vi "Line_Line_Intersection2D_Test_PN.vi"(3 "2D Dir. Vect. of Line 2 (not unit)":dbl[](array[numeric])=[0.0, 0.0], 4 "2D Dir. Vect. of Line 1 (not unit)":dbl[](array[numeric])=[0.0, 0.0], 5 "2D Point on Line 2":dbl[](array[numeric])=[0.0, 0.0], 6 "2D Point on Line 1":dbl[](array[numeric])=[0.0, 0.0]) -> (0 "s2":dbl, 1 "s1":dbl, 2 "Lines Intersect":bool)   [LabVIEW 2011]
panel:
  in  "1+eps":dbl=1.000000000001 format="%#_16f"
  in  "-eps":dbl=-1e-12 format="%#_16f"
  # "The direction vectors must not be unit vectors.\nThe input points must be the tail points of the associated line vectors.\ns1 represents the distance from the start point of line 1 to the intersection point.\ns2 represents the distance from the start point of line 2 to the intersection point."
  # "Paul Nathan 04/03/10"
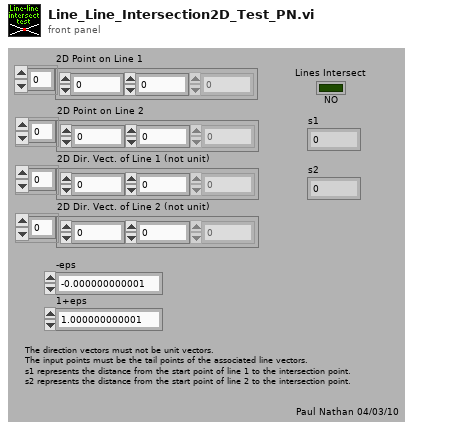
[diagram p1: front panel]
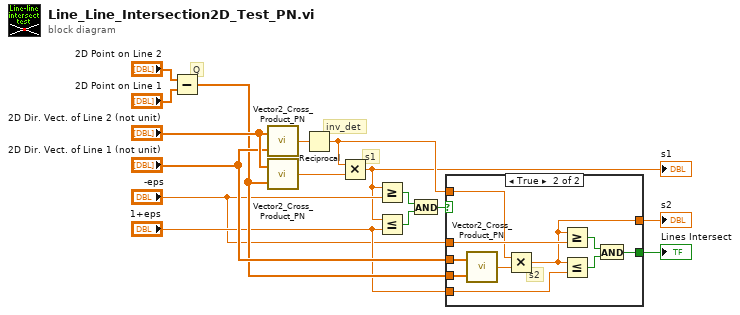
[diagram p0: block diagram]
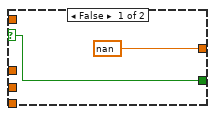
[diagram p2: hidden frame]
diagram:
  # "s1"
  # "inv_det"
  # "Q"
  n1 = Subtract(x="2D Point on Line 2", y="2D Point on Line 1") -> (x-y=w7:dbl[])
  n2 = call "Vector2_Cross_Product_PN.vi"("V (2D)"="2D Dir. Vect. of Line 1 (not unit)", "U (2D)"="2D Dir. Vect. of Line 2 (not unit)") -> ("U X V (2D)"=w14:dbl)
  n3 = call "Vector2_Cross_Product_PN.vi"("V (2D)"=w7, "U (2D)"="2D Dir. Vect. of Line 2 (not unit)") -> ("U X V (2D)"=w12:dbl)
  n4 = Reciprocal(x=w14) -> (1/x=w3:dbl)
  n5 = Multiply(x=w3, y=w12) -> (x*y=w1:dbl)
  "s1" <- w1
  n6 = Greater Or Equal?(x=w1, y="-eps") -> (x >= y?=w11:bool)
  n7 = Less Or Equal?(x=w1, y="1+eps") -> (x <= y?=w10:bool)
  n8 = And(x=w11, y=w10) -> (x .and. y?=w9:bool)
  n9 = case shown="True" w9 {
    selector: w9 -> [w17 _]
    tunnel: "2D Dir. Vect. of Line 1 (not unit)" -> [_ w28]
    tunnel: w7 -> [_ w27]
    tunnel: "-eps" -> [_ w23]
    tunnel: "1+eps" -> [_ w22]
    tunnel: [w17 w21] -> w5
    tunnel: [nan w20] -> w4
    tunnel: w3 -> [_ w19]
    frame False {
    }
    frame True {
      # "s2"
      n10 = call "Vector2_Cross_Product_PN.vi"("V (2D)"=w27, "U (2D)"=w28) -> ("U X V (2D)"=w26:dbl)
      n11 = Multiply(x=w19, y=w26) -> (x*y=w20:dbl)
      n12 = Greater Or Equal?(x=w20, y=w23) -> (x >= y?=w24:bool)
      n13 = Less Or Equal?(x=w20, y=w22) -> (x <= y?=w25:bool)
      n14 = And(x=w24, y=w25) -> (x .and. y?=w21:bool)
    }
  }
  "Lines Intersect" <- w5
  "s2" <- w4
